vi "WriteControlHeader.vi"(6 "ErrorIn":errorcluster, 8 "RobotOffsets":dbl[](array[numeric]), 9 "ControlParams":T1={"Kx"=30.0, "Ky"=1.0, "Kt"=50.0, "d"=0.07, "Ks"=80.0, "MinV"=0.0, "MaxV"=1000.0, "Ka"=0.07}, 10 "RobotGains":T2, 11 "ControlStream":refnum<file>) -> (0 "ErrorOut":errorcluster, 3 "ControlStreamOut":refnum<file>)   [LabVIEW 2013]
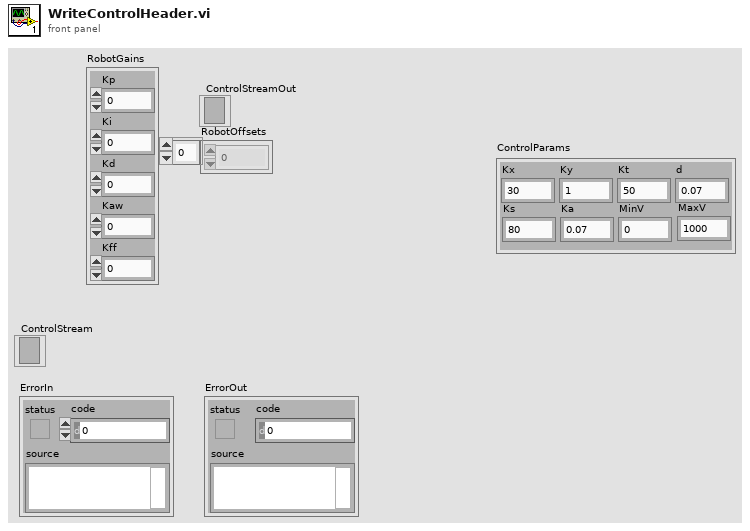
[diagram p1: front panel]
types:
  T1 = cluster{"Kx":dbl, "Ky":dbl, "Kt":dbl, "d":dbl, "Ks":dbl, "MinV":dbl, "MaxV":dbl, "Ka":dbl}
  T2 = cluster{"Kp":u16, "Ki":u16, "Kd":u16, "Kaw":u16, "Kff":u16}
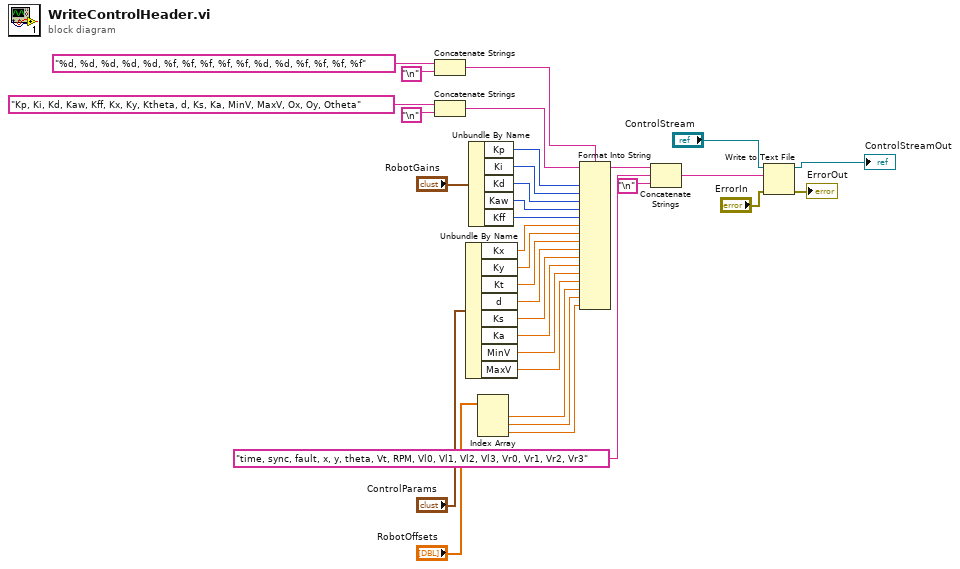
[diagram p0: block diagram]
diagram:
  n1 = Concatenate Strings("%d, %d, %d, %d, %d, %f, %f, %f, %f, %f, %d, %d, %f, %f, %f, %f" ("format string"), "\n") -> (w25:string)
  n2 = Concatenate Strings("Kp, Ki, Kd, Kaw, Kff, Kx, Ky, Ktheta, d, Ks, Ka, MinV, MaxV, Ox, Oy, Otheta" ("initial string"), "\n") -> (w22:string)
  n3 = Unbundle By Name("ControlParams") -> ("Kx"=w8:dbl, "Ky"=w7:dbl, "Kt"=w6:dbl, "d"=w5:dbl, "Ks"=w4:dbl, "Ka"=w3:dbl, "MinV"=w2:dbl, "MaxV"=w1:dbl)
  n4 = Unbundle By Name("RobotGains") -> ("Kp"=w13:u16, "Ki"=w12:u16, "Kd"=w11:u16, "Kaw"=w10:u16, "Kff"=w9:u16)
  n5 = Index Array(array="RobotOffsets") -> (element #1=w18:dbl, element #2=w17:dbl, element #3=w16:dbl)  [unwired: 3 in]
  n6 = Format Into String(format string=w25, initial string=w22, w13, w12, w11, w10, w9, w8, w7, w6, w5, w4, w3, w2, w1, w18, w17, w16) -> (resulting string=w28:string)  [unwired: 1 in, 1 out]
  n7 = Concatenate Strings(w28, "time, sync, fault, x, y, theta, Vt, RPM, Vl0, Vl1, Vl2, Vl3, Vr0, Vr1, Vr2, Vr3" ("initial string"), "\n") -> (w29:string)
  n8 = Write to Text File(file (use dialog)="ControlStream", text=w29, error in="ErrorIn") -> (refnum out=→"ControlStreamOut":refnum<file>, error out=→"ErrorOut":errorcluster)  [unwired: 1 in, 1 out]
